vi "HEWH RLT Check Cutout Delay.vi"(6 "Delay After Cutout (sec)":dbl=1.0, 7 "Use Cutout Delay":bool, 8 "Error In":errorcluster, 10 "Start Draw":bool, 11 "Heat Source ON (1=ON)":bool) -> (0 "Error Out":errorcluster, 3 "Full Cutout?":bool)   [LabVIEW 2016]
panel:
  out "Cut In Timer (Over)":bool
  out "Cut Out Timer (Over)":bool
  out "Elapsed Time (sec) 2":dbl format="%.2f"
  out "Elapsed Time (sec)":dbl format="%.2f"
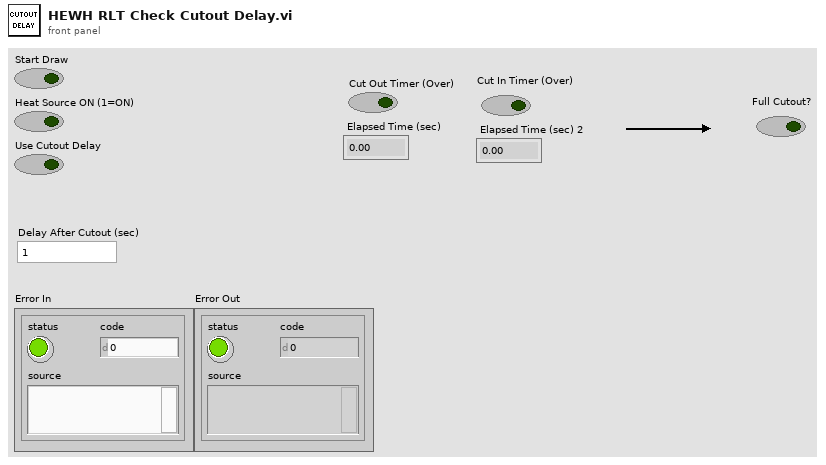
[diagram p1: front panel]
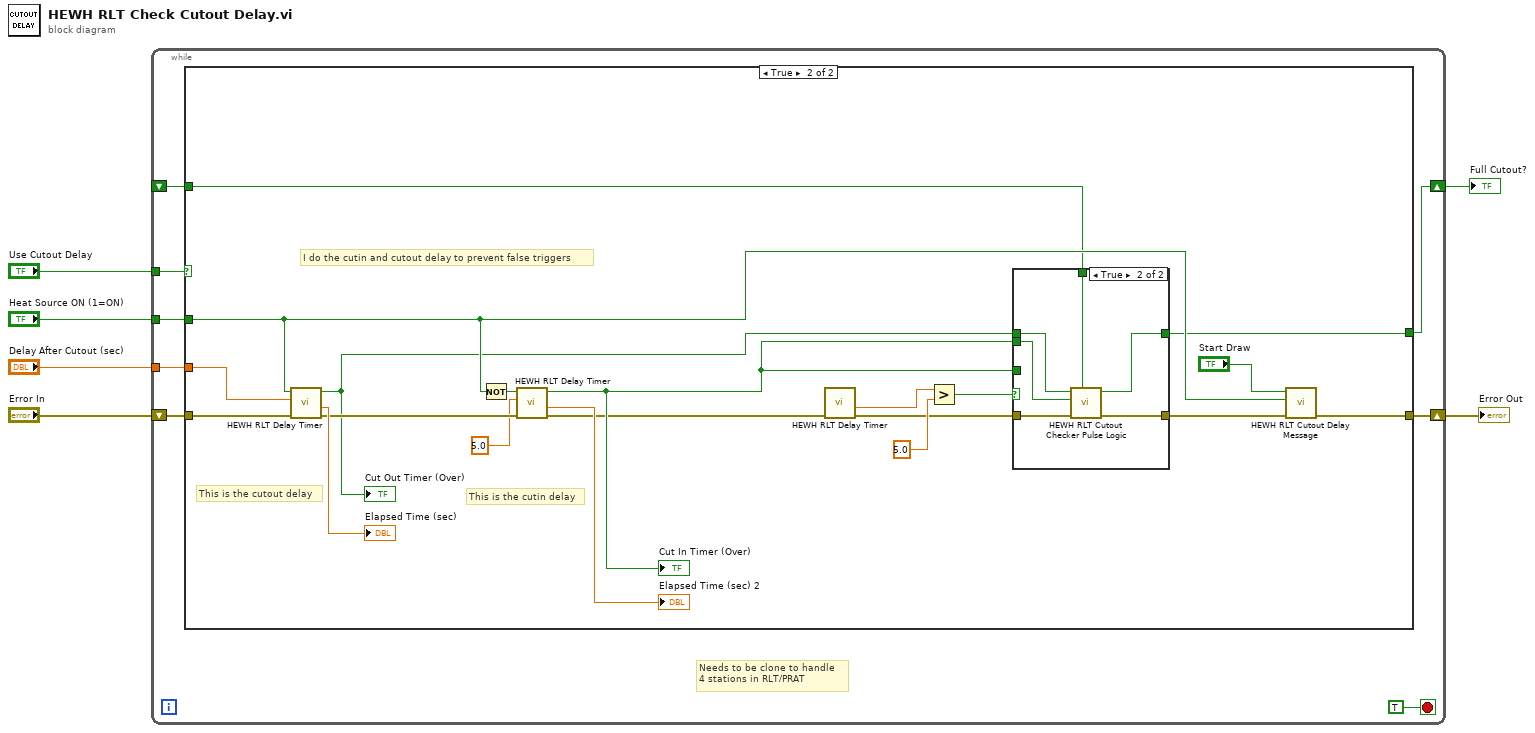
[diagram p0: block diagram]
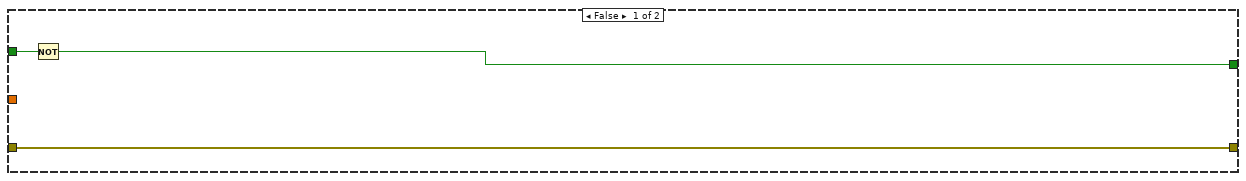
[diagram p2: hidden frame]
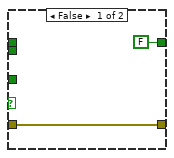
[diagram p3: hidden frame]
diagram:
  n1 = while {
    tunnel: "Use Cutout Delay" -> [w14]
    tunnel: "Delay After Cutout (sec)" -> [w10]
    shift-right: [w12] -> w4
    shift-left: "Error In" -> [w11]
    shift-right: [w13] -> w5
    shift-left: _ -> [w7]
    tunnel: "Heat Source ON (1=ON)" -> [w8]
    stop <- TRUE stop-if-true
    # "Needs to be clone to handle\n4 stations in RLT/PRAT"
    n2 = case shown="True" w14 {
      tunnel: [w16 w25] -> w13
      tunnel: w11 -> [w17 w35]
      tunnel: [w17 w34] -> w12
      tunnel: w8 -> [w15 w28]
      tunnel: w10 -> [_ w36]
      tunnel: w7 -> [_ w18]
      frame False {
        n3 = Not(x=w15) -> (.not. x?=w16:bool)
      }
      frame True {
        # "This is the cutout delay"
        # "This is the cutin delay"
        # "I do the cutin and cutout delay to prevent false triggers"
        n4 = call "HEWH RLT Delay Timer.vi"("Error In"=w35, "Delay After Cutout (sec)"=w36, "Heat Source ON (1=ON)"=w28) -> ("Error Out"=w32:errorcluster, "Elapsed Time (sec)"=→"Elapsed Time (sec)":dbl, "Delay is Over"=w27:bool)  [unwired: 6 in]
        "Cut Out Timer (Over)" <- w27
        n5 = Not(x=w28) -> (.not. x?=w31:bool)
        n6 = call "HEWH RLT Delay Timer.vi"("Error In"=w32, "Delay After Cutout (sec)"=5.0, "Heat Source ON (1=ON)"=w31) -> ("Error Out"=w24:errorcluster, "Elapsed Time (sec)"=→"Elapsed Time (sec) 2":dbl, "Delay is Over"=w26:bool)  [unwired: 6 in]
        "Cut In Timer (Over)" <- w26
        n7 = call "HEWH RLT Delay Timer.vi"("Error In"=w24) -> ("Error Out"=w20:errorcluster, "Elapsed Time (sec)"=w23:dbl)  [unwired: 8 in, 1 out]
        n8 = Greater?(x=w23, y=5.0) -> (0:w21:bool)
        n9 = case shown="True" w21 {
          tunnel: w26 -> [_ _]
          tunnel: [FALSE w43] -> w25
          tunnel: w27 -> [_ w45]
          tunnel: w26 -> [_ w44]
          tunnel: w20 -> [w38 w42]
          tunnel: [w38 w41] -> w19
          tunnel: w18 -> [_ w40]
          frame False {
          }
          frame True {
            n10 = call "HEWH RLT Cutout Checker Pulse Logic.vi"("Previous Full Cutout Value"=w40, "Error In"=w42, "Cut In Timer (Over)"=w44, "Cut Out Timer (Over)"=w45) -> ("Error Out"=w41:errorcluster, "Full Cutout?"=w43:bool)  [unwired: 6 in]
          }
        }
        n11 = call "HEWH RLT Cutout Delay Message.vi"("error in (no error)"=w19, "Heat Source ON (1=ON)"=w28, "Start Draw"="Start Draw") -> ("error out"=w34:errorcluster)  [unwired: 8 in]
      }
    }
  }
  "Full Cutout?" <- w5
  "Error Out" <- w4
